vi "Sysfs GPIO Blinking LED.vi"() -> ()   [LabVIEW 2014]
uses:
  vi.lib/Q-WaveSystems/QwaveSys Raspberry Pi for LabVIEW Home-Education/Sysfs_GPIO/RPi GPIO.ctl
  vi.lib/Q-WaveSystems/QwaveSys Raspberry Pi for LabVIEW Home-Education/QwaveSys Raspberry Pi Library.lvlib
panel:
  in  "Delay (ms)":u32=1000
  in  "Rpi.GPIO":T1=7 items=["GPIO2 (P1_3-SDA)"=2, "GPIO3 (P1_5-SCL)"=3, "GPIO4 (P1_7)"=4, "GPIO17 (P1_11)"=17, "GPIO27 (P1_13)"=27, "GPIO22 (P1_15)"=22, "GPIO10 (P1_19-MOSI)"=10, "GPIO9 (P1_21-MISO)"=9, "GPIO11 (P1_23SCLK)"=11, "GPIO5 (P1_29)"=5, "GPIO6 (P1_31)"=6, "GPIO13 (P1_33-PWM1)"=13, "GPIO19 (P1_35)"=19, "GPIO26 (P1_37)"=26, "GPIO14 (P1_8-UART-Tx)"=14, "GPIO15 (P1_10-UART-Rx)"=15, "GPIO18 (P1_12)"=18, "GPIO23 (P1_16)"=23, "GPIO24 (P1_18)"=24, "GPIO25 (P1_22)"=25, "GPIO8 (P1_24-CE0)"=8, "GPIO7 (P1_26-CE1)"=7, "GPIO12 (P1_32-PWM0)"=12, "GPIO16 (P1_36)"=16, "GPIO20 (P1_38)"=20, "GPIO21 (P1_40)"=21]
  out "LED":bool
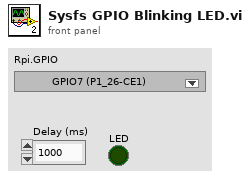
[diagram p1: front panel]
types:
  T1 = typedef "QwaveSys Raspberry Pi Library.lvlib/RPi GPIO.ctl" = u8
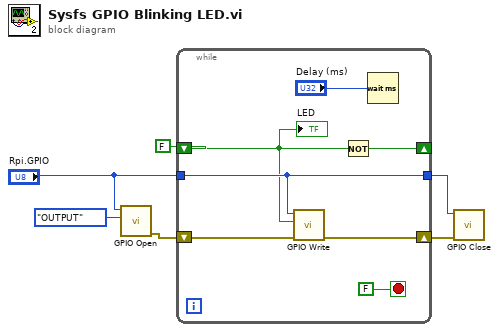
[diagram p0: block diagram]
diagram:
  n1 = call "GPIO Open.vi"("mode"=enum16{"OUTPUT", "INPUT"}."OUTPUT", "Rpi.GPIO"="Rpi.GPIO") -> ("error out"=w5:errorcluster)  [unwired: 9 in]
  n2 = while {
    shift-right: [w9] -> w4
    shift-left: w5 -> [w10]
    tunnel: [w8] -> w1
    tunnel: "Rpi.GPIO" -> [w8]
    shift-right: [w12] -> _
    shift-left: FALSE -> [w7]
    stop <- FALSE stop-if-true
    n3 = call "GPIO Write.vi"("error in (no error)"=w10, "status"=w7, "Rpi.GPIO"=w8) -> ("error out"=w9:errorcluster)  [unwired: 8 in]
    n4 = Not(x=w7) -> (.not. x?=w12:bool)
    n5 = Wait (ms)(milliseconds to wait="Delay (ms)") -> ()  [unwired: 1 out]
    "LED" <- w7
  }
  n6 = call "GPIO Close.vi"("error in (no error)"=w4, "Rpi.GPIO"=w1) -> ()  [unwired: 9 in, 1 out]
